vi "LU20_krio_main__.vi"() -> ()   [LabVIEW 2015]
doc: "Программа мониторинга температуры ОГ-1000"
uses:
  <vilib>/NI/Modbus Library/API/Master/Modbus Master.lvclass
  <vilib>/Utility/error.llb/DialogType.ctl
panel:
  out "Связь с блоком":bool
  in  "Tab Control":enum32{"ИЗМЕРЕНИЯ [ K ]", "НАСТРОЙКИ"}(tab)
  out "R2":dbl format="%.2f"
  out "R1":dbl format="%.2f"
  in  "2_ch_visible":bool=TRUE
  in  "1_ch_visible":bool=TRUE
  out "T2":dbl format="%.2f"
  out "T1":dbl format="%.2f"
  out "Путь к файлу с коэф.":path
  in  "Пароль":string
  in  "настр. коэфф.":bool caption="Disconn"
  in  "Coeff_cl_ch2":T1={"k1"=31.9101907935109921, "k2"=-399.867376562207937, "k3"=2119.32627579197288, "k4"=-5531.15447566658258, "k5"=7772.21873644739389, "k6"=-5292.23886113613844, "k7"=1613.2211984321475, "R0"=1613.2211984321475} caption="T2" {"R0" format="%#_16g"; "k7" format="%#_16g"; "k6" format="%#_16g"; "k5" format="%#_16g"; "k4" format="%#_16g"; "k3" format="%#_16g"; "k2" format="%#_16g"; "k1" format="%#_16g"}
  in  "load_coeff.":bool caption="Disconn"
  in  "save_coeff.":bool caption="Disconn"
  in  "xScale -":bool
  in  "xScale +":bool
  out "мин.":string="1"
  in  "Добавить время":dbl(ring)=300.0 items=["10 сек."=10.0, "1 мин."=60.0, "5 мин."=300.0, "20 мин."=1200.0]
  out "часы":string="0"
  out "сек.":string="0"
  in  "stop":bool
  in  "Coeff_cl_ch1":T1 caption="T1" {"R0" format="%#_16g"; "k7" format="%#_16g"; "k6" format="%#_16g"; "k5" format="%#_16g"; "k4" format="%#_16g"; "k3" format="%#_16g"; "k2" format="%#_16g"; "k1" format="%#_16g"}
  in  "GraphLookB":bool
  in  "Т min":dbl=4.0 min=-10.0 max=350.0 step=0.1
  in  "Т max":dbl=350.0 min=2.0 max=500.0 step=0.1
  in  "Autoscale":bool=TRUE
  in  "IP":string
  in  "Порт":u16
  out "Сутки":string
  in  "Запись в файл":bool
  out "Path":string
  out "File header exist?":bool caption="Disconn"
  in  "ADC_dyn_range":T2(ring)=enum."± 0.625 В"
  out "refnum out":refnum<file>
  out "Graphs T":dynamicdata(graph) caption="ИЗМЕРЕНИЯ ТЕМПЕРАТУРЫ, К"
  out "Связь":refnum<class "Modbus Master.lvclass">
  in  "Buf_size":u8=1 min=1 max=128
  in  "SPS":T3(ring)
  out "Расположение файла":path
  # "Соед."
  # "K"
  # "K"
  # "Ом"
  # "Ом"
  # ":"
  # ":"
  # "id 102"
  # "Шкала Т"
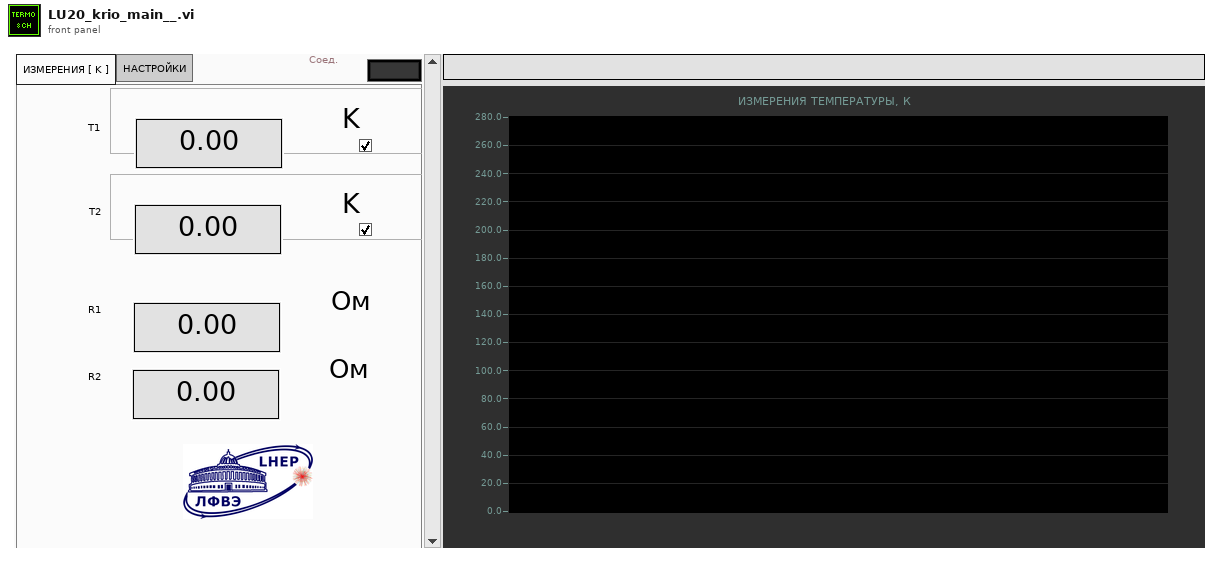
[diagram p1: front panel]
types:
  T1 = cluster{"k1":ext, "k2":ext, "k3":ext, "k4":ext, "k5":ext, "k6":ext, "k7":ext, "R0":ext}
  T2 = enum16{"± 5 В", "± 2.5 В", "± 1.25 В", "± 0.625 В", "± 312.5 мВ", "± 156.25 мВ", "± 78.125 мВ"}
  T3 = enum16{"2,5 SPS", "5 SPS", "10 SPS", "25 SPS", "50 SPS", "100 SPS", "500 SPS", "1 kSPS"}
  T4 = typedef "DialogType.ctl" = u16
  T5 = enum8{"Enabled", "Disabled", "Disabled and Grayed Out"}
  T6 = typedef "LVDateTimeRec.ctl" = cluster{"fractional second":dbl, "second":i32, "minute":i32, "hour":i32, "day of month":i32, "month":i32, "year":i32, "day of week":i32, "day of year":i32, "DST":i32}
  T7 = enum16{"open", "replace", "create", "open or create", "replace or create", "replace or create with confirmation"}
  T8 = cluster{"k1":ext, "k2":ext, "k3":ext, "k4":ext, "k5":ext, "k6":ext, "k7":ext, "R":ext}
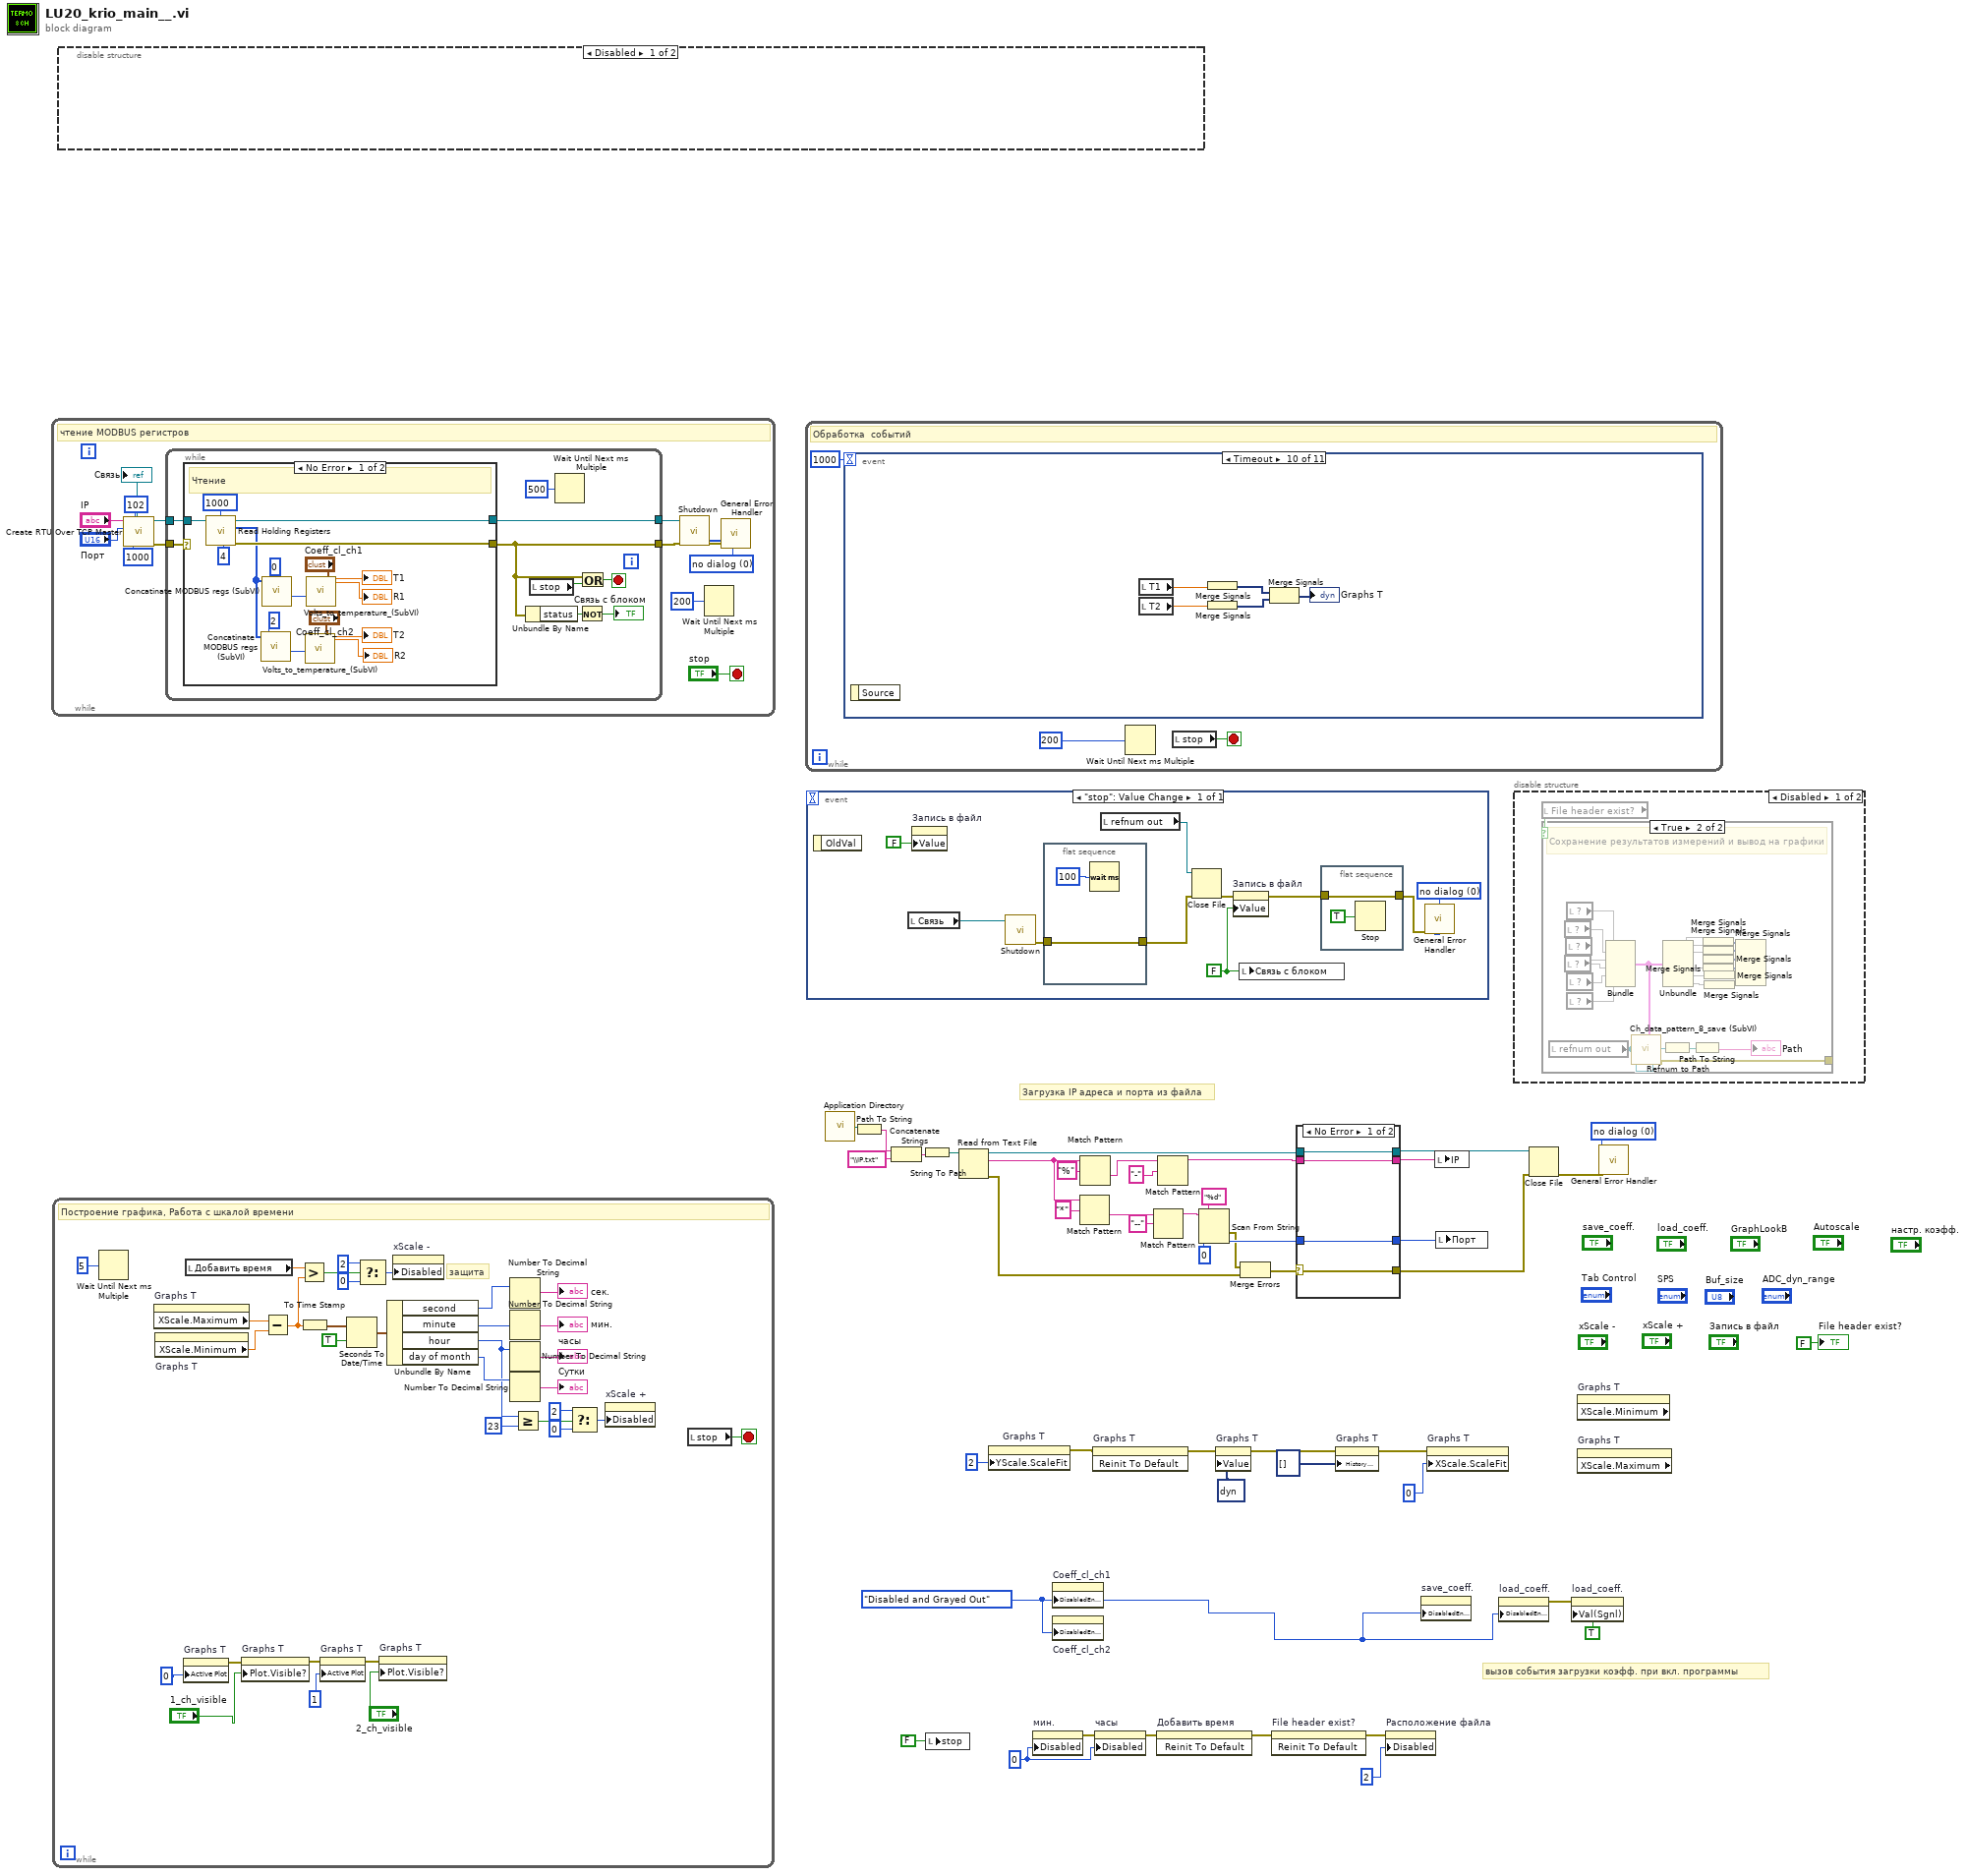
[diagram p0: block diagram]
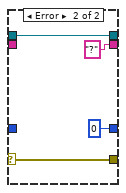
[diagram p2: hidden frame]
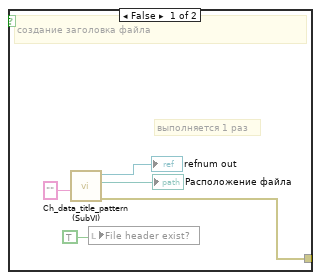
[diagram p4: hidden frame]
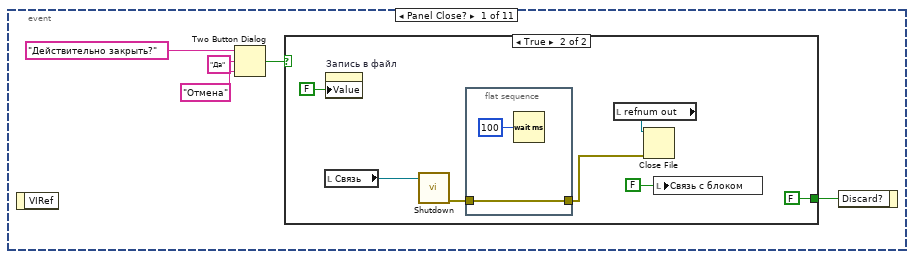
[diagram p6: hidden frame]
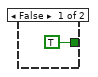
[diagram p7: hidden frame]
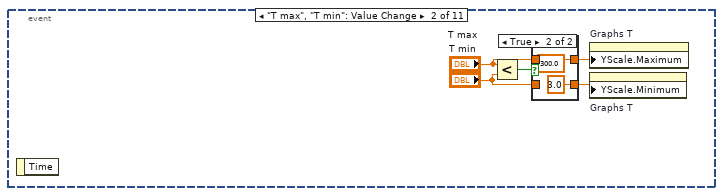
[diagram p8: hidden frame]
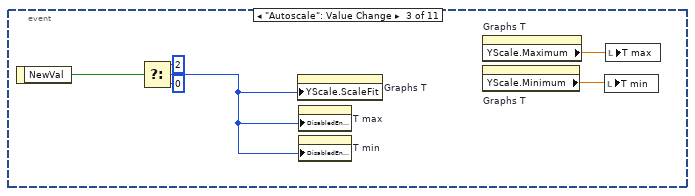
[diagram p10: hidden frame]
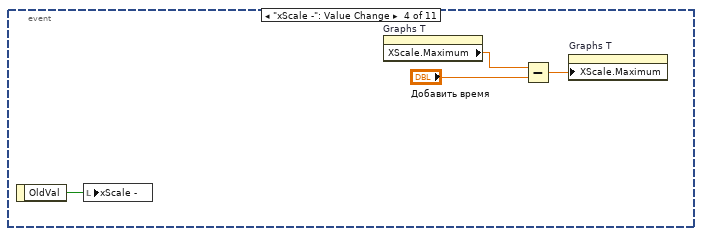
[diagram p11: hidden frame]
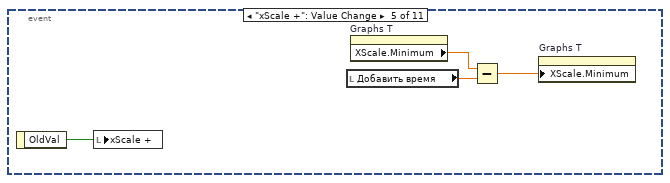
[diagram p12: hidden frame]
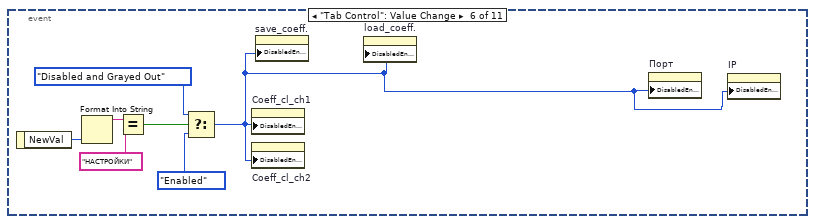
[diagram p13: hidden frame]
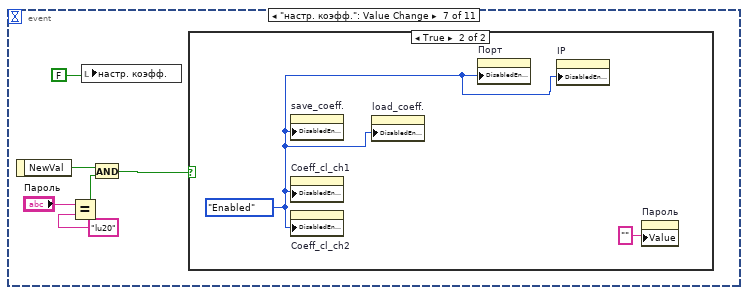
[diagram p14: hidden frame]
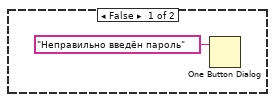
[diagram p15: hidden frame]
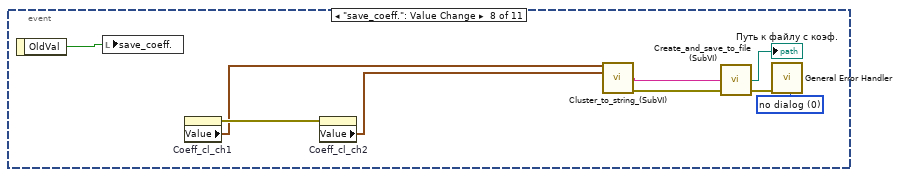
[diagram p16: hidden frame]
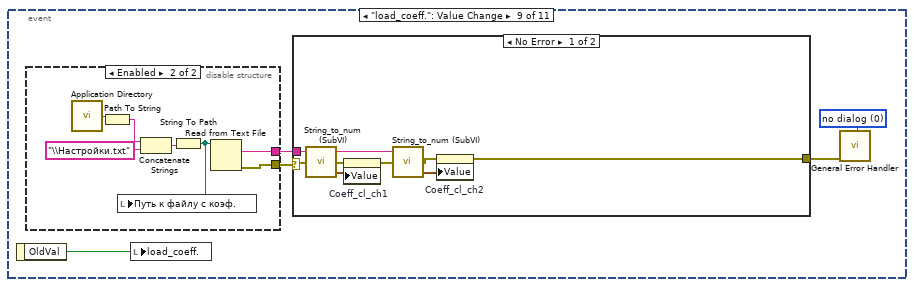
[diagram p17: hidden frame]
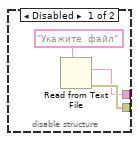
[diagram p18: hidden frame]
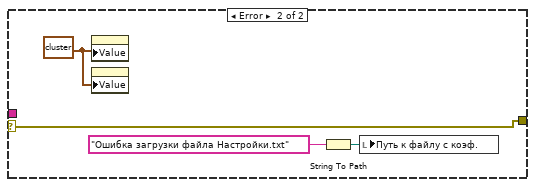
[diagram p19: hidden frame]
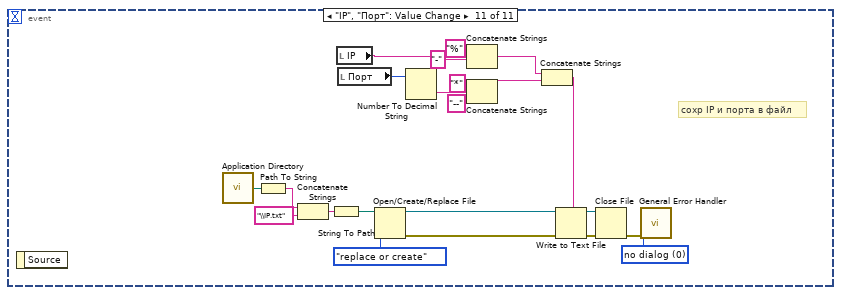
[diagram p20: hidden frame]
diagram:
  w10 = T4 0 items=["no dialog", "OK message", "continue or stop message", "OK message + warnings", "continue/stop + warnings"] ("type of dialog (OK msg:1)")
  w38 = T5."Disabled and Grayed Out" ("Disabled")
  w45 = u8 0 ("Disabled")
  # "Загрузка IP адреса и порта из файла"
  # "вызов события загрузки коэфф. при вкл. программы"
  n1 = while {
    stop <- "stop" stop-if-true
    w47 = T4 0 items=["no dialog", "OK message", "continue or stop message", "OK message + warnings", "continue/stop + warnings"] ("type of dialog (OK msg:1)")
    # "чтение MODBUS регистров"
    n2 = call "Create RTU Over TCP Master.vi"("unit ID"=u8 102 ("ID"), "connect timeout ms"=1000, "port (502)"="Порт", "address"="IP") -> ("error out"=w51:errorcluster, "TCP master instance"=w52:refnum<class "Modbus Master.lvclass">)  [unwired: 6 in]
    "Связь" <- w52
    n3 = while {
      tunnel: w52 -> [w67]
      tunnel: w51 -> [w66]
      tunnel: [w60] -> w50
      tunnel: [w65] -> w49
      stop <- w63 stop-if-true
      n4 = case shown="No Error" w66 {
        selector: w66 -> [_ w84]
        tunnel: w67 -> [w81 w85]
        tunnel: [w78 w84] -> w60
        tunnel: [w80 w85] -> w65
        frame No Error {
          # "Чтение"
          n5 = call-dynamic "Read Holding Registers.vi"("number of inputs"=u16 4, "starting address"=u16 1000, "Modbus master in"=w81) -> ("error out"=w78:errorcluster, "register values"=w72:u16[], "Modbus master out"=w80:refnum<class "Modbus Master.lvclass">)  [unwired: 6 in]
          n6 = call "Concatinate MODBUS regs (SubVI).vi"("LSB reg num"=u16 2, "registers array in"=w72) -> ("register data"=w74:i32)  [unwired: 8 in, 1 out]
          n7 = call "Concatinate MODBUS regs (SubVI).vi"("LSB reg num"=u16 0, "registers array in"=w72) -> ("register data"=w76:i32)  [unwired: 8 in, 1 out]
          n8 = call "Volts_to_temperature_(SubVI).vi"("Resistance"=w74, "koeff. cluster"="Coeff_cl_ch2") -> ("T solvation"=→"T2":dbl, "meas_voltage"=→"R2":dbl)  [unwired: 21 in, 3 out]
          n9 = call "Volts_to_temperature_(SubVI).vi"("Resistance"=w76, "koeff. cluster"="Coeff_cl_ch1") -> ("T solvation"=→"T1":dbl, "meas_voltage"=→"R1":dbl)  [unwired: 21 in, 3 out]
        }
        frame Error {
        }
      }
      n10 = Unbundle By Name(w60) -> ("status"=w62:bool)
      n11 = local read "stop"() -> (w64:bool)
      n12 = Wait Until Next ms Multiple(millisecond multiple=u32 500) -> ()  [unwired: 1 out]
      n13 = Not(x=w62) -> (.not. x?=→"Связь с блоком":bool)
      n14 = Or(x=w60, y=w64) -> (x .or. y?=w63:bool)
    }
    n15 = call-dynamic "Shutdown.vi"("error in"=w50, "Modbus master in"=w49) -> ("error out"=w48:errorcluster)  [unwired: 9 in]
    n16 = Wait Until Next ms Multiple(millisecond multiple=u32 200) -> ()  [unwired: 1 out]
    n17 = call <vilib>:"General Error Handler.vi"("type of dialog (OK msg:1)"=w47, "error in (no error)"=w48) -> ()  [unwired: 1 in, 13 out]
  }
  n18 = while {
    stop <- w118 stop-if-true
    # "защита"
    # "Построение графика, Работа с шкалой времени"
    n19 = Wait Until Next ms Multiple(millisecond multiple=u32 5) -> ()  [unwired: 1 out]
    n20 = property on="Graphs T" class="WFChart (strict)"() -> ("XScale.Maximum"=w94:dbl)  [unwired: 2 in, 2 out]
    n21 = property on="Graphs T" class="WFChart (strict)"() -> ("XScale.Minimum"=w93:dbl)  [unwired: 2 in, 2 out]
    n22 = property on="Graphs T" class="WFChart (strict)"("Active Plot"=u32 0) -> (error out=w86:errorcluster)  [unwired: 2 in, 1 out]
    n23 = local read "Добавить время"() -> (w117:dbl)
    n24 = property on="Graphs T" class="WFChart (strict)"(error in=w86, "Plot.Visible?"="1_ch_visible") -> (error out=w91:errorcluster)  [unwired: 1 in, 1 out]
    n25 = Subtract(x=w94, y=w93) -> (x-y=w107:dbl)
    n26 = Greater?(x=w117, y=w107) -> (0:w100:bool)
    n27 = To Time Stamp(1:w107) -> (0:w115:timestamp)
    n28 = property on="Graphs T" class="WFChart (strict)"(error in=w91, "Active Plot"=u32 1) -> (error out=w89:errorcluster)  [unwired: 1 in, 1 out]
    n29 = Seconds To Date/Time(time stamp (now)=w115, to UTC (F)=TRUE) -> (date time rec=w114:T6)
    n30 = Select(t=u8 2 ("Disabled"), s=w100, f=u8 0 ("Disabled")) -> (s? t:f=w103:u8)
    n31 = property on="Graphs T" class="WFChart (strict)"(error in=w89, "Plot.Visible?"="2_ch_visible") -> ()  [unwired: 1 in, 2 out]
    n32 = Unbundle By Name(w114) -> ("second"=w113:i32, "minute"=w112:i32, "hour"=w105:i32, "day of month"=w111:i32)
    n33 = property on="xScale -" class="Bool (strict)"("Disabled"=w103) -> ()  [unwired: 2 in, 2 out]
    n34 = Number To Decimal String(number=w113) -> (decimal integer string=→"сек.":string)  [unwired: 1 out]
    n35 = Number To Decimal String(number=w112) -> (decimal integer string=→"мин.":string)  [unwired: 1 out]
    n36 = Number To Decimal String(number=w105) -> (decimal integer string=→"часы":string)  [unwired: 1 out]
    n37 = Number To Decimal String(number=w111) -> (decimal integer string=→"Сутки":string)  [unwired: 1 out]
    n38 = Greater Or Equal?(x=w105, y=23) -> (x >= y?=w96:bool)
    n39 = Select(t=u8 2 ("Disabled"), s=w96, f=u8 0 ("Disabled")) -> (s? t:f=w99:u8)
    n40 = property on="xScale +" class="Bool (strict)"("Disabled"=w99) -> ()  [unwired: 2 in, 2 out]
    n41 = local read "stop"() -> (w118:bool)
  }
  n42 = disable-structure shown="Disabled" {
    frame Disabled {
    }
    frame Enabled {
    }
  }
  n43 = while {
    stop <- w120 stop-if-true
    # "Обработка  событий"
    n44 = event shown="[9] Timeout" {
      selector: _ -> [_ _ _ _ _ _ _ _ _ _ _]
      dyn-events: _ -> [_ _ _ _ _ _ _ _ _ _ _]
      timeout: 1000 -> [_ _ _ _ _ _ _ _ _ _ _]
      event Panel Close? {
        n45 = event-data() -> ()  [unwired: 2 out]
        n46 = Two Button Dialog(message="Действительно закрыть?", 1:"Отмена" ("T button name (\"OK\")"), 2:"Да" ("T button name (\"OK\")")) -> (T button?=w126:bool)
        n47 = case shown="True" w126 {
          tunnel: [TRUE ("Discard?") FALSE ("Discard?")] -> w122
          frame False {
          }
          frame True {
            n48 = local read "Связь"() -> (w131:refnum<class "Modbus Master.lvclass">)
            n49 = property on="Запись в файл" class="Bool (strict)"("Value"=FALSE ("Запись в файл")) -> ()  [unwired: 2 in, 2 out]
            n50 = call-dynamic "Shutdown.vi"("Modbus master in"=w131) -> ("error out"=w130:errorcluster)  [unwired: 10 in]
            n51 = flat-sequence {
              tunnel: w130 -> [w135]
              tunnel: [w135] -> w129
              frame #0 {
                n52 = Wait (ms)(milliseconds to wait=u32 100) -> ()  [unwired: 1 out]
              }
            }
            n53 = local read "refnum out"() -> (w133:refnum<file>)
            n54 = Close File(refnum=w133, error in=w129) -> ()  [unwired: 2 out]
            n55 = local write "Связь с блоком"(FALSE ("Связь с блоком 4")) -> ()
          }
        }
        n56 = event-data("Discard?"=w122) -> ()  [unwired: 1 in, 1 out]
      }
      event "Т max", "Т min": Value Change {
        n57 = event-data() -> ()  [unwired: 2 out]
        n58 = Less?(x="Т max", y="Т min") -> (x < y?=w141:bool)
        n59 = case shown="True" w141 {
          tunnel: [w142 300.0 ("x+1")] -> w139
          tunnel: [w143 3.0 ("x+1")] -> w140
          tunnel: "Т max" -> [w142 _]
          tunnel: "Т min" -> [w143 _]
          frame False {
          }
          frame True {
          }
        }
        n60 = property on="Graphs T" class="WFChart (strict)"("YScale.Maximum"=w139) -> ()  [unwired: 2 in, 2 out]
        n61 = property on="Graphs T" class="WFChart (strict)"("YScale.Minimum"=w140) -> ()  [unwired: 2 in, 2 out]
      }
      event "Autoscale": Value Change {
        n62 = event-data() -> ("NewVal"=w146:bool)  [unwired: 1 out]
        n63 = Select(t=u8 2 ("Y Scale.Scale Fit"), s=w146, f=u8 0 ("Y Scale.Scale Fit")) -> (s? t:f=w149:u8)
        n64 = property on="Graphs T" class="WFChart (strict)"("YScale.ScaleFit"=w149) -> ()  [unwired: 2 in, 2 out]
        n65 = property on="Т max" class="DigNum (strict)"("DisabledEnum"=w149) -> ()  [unwired: 2 in, 2 out]
        n66 = property on="Т min" class="DigNum (strict)"("DisabledEnum"=w149) -> ()  [unwired: 2 in, 2 out]
        n67 = property on="Graphs T" class="WFChart (strict)"() -> ("YScale.Maximum"=w151:dbl)  [unwired: 2 in, 2 out]
        n68 = property on="Graphs T" class="WFChart (strict)"() -> ("YScale.Minimum"=w150:dbl)  [unwired: 2 in, 2 out]
        n69 = local write "Т min"(w150) -> ()
        n70 = local write "Т max"(w151) -> ()
      }
      event "xScale -": Value Change {
        n71 = event-data() -> ("OldVal"=w155:bool)  [unwired: 1 out]
        n72 = local write "xScale -"(w155) -> ()
        n73 = property on="Graphs T" class="WFChart (strict)"() -> ("XScale.Maximum"=w153:dbl)  [unwired: 2 in, 2 out]
        n74 = Subtract(x=w153, y="Добавить время") -> (x-y=w152:dbl)
        n75 = property on="Graphs T" class="WFChart (strict)"("XScale.Maximum"=w152) -> ()  [unwired: 2 in, 2 out]
      }
      event "xScale +": Value Change {
        n76 = event-data() -> ("OldVal"=w159:bool)  [unwired: 1 out]
        n77 = local write "xScale +"(w159) -> ()
        n78 = local read "Добавить время"() -> (w158:dbl)
        n79 = property on="Graphs T" class="WFChart (strict)"() -> ("XScale.Minimum"=w157:dbl)  [unwired: 2 in, 2 out]
        n80 = Subtract(x=w157, y=w158) -> (x-y=w156:dbl)
        n81 = property on="Graphs T" class="WFChart (strict)"("XScale.Minimum"=w156) -> ()  [unwired: 2 in, 2 out]
      }
      event "Tab Control": Value Change {
        n82 = event-data() -> ("NewVal"=w166:enum32{"ИЗМЕРЕНИЯ [ K ]", "НАСТРОЙКИ"})  [unwired: 1 out]
        n83 = Format Into String(w166) -> (resulting string=w165:string)  [unwired: 3 in, 1 out]
        n84 = Equal?(x=w165, y="НАСТРОЙКИ") -> (x = y?=w163:bool)
        n85 = Select(t=T5."Disabled and Grayed Out" ("Disabled"), s=w163, f=T5."Enabled" ("Disabled")) -> (s? t:f=w160:T5)
        n86 = property on="Coeff_cl_ch1" class="Clust (strict)"("DisabledEnum"=w160) -> ()  [unwired: 2 in, 2 out]
        n87 = property on="Coeff_cl_ch2" class="Clust (strict)"("DisabledEnum"=w160) -> ()  [unwired: 2 in, 2 out]
        n88 = property on="save_coeff." class="Bool (strict)"("DisabledEnum"=w160) -> ()  [unwired: 2 in, 2 out]
        n89 = property on="load_coeff." class="Bool (strict)"("DisabledEnum"=w160) -> ()  [unwired: 2 in, 2 out]
        n90 = property on="Порт" class="DigNum (strict)"("DisabledEnum"=w160) -> ()  [unwired: 2 in, 2 out]
        n91 = property on="IP" class="Str"("DisabledEnum"=w160) -> ()  [unwired: 2 in, 2 out]
      }
      event "настр. коэфф.": Value Change {
        n92 = event-data() -> ("NewVal"=w172:bool)  [unwired: 1 out]
        n93 = Equal?(x="Пароль", y="lu20") -> (x = y?=w169:bool)
        n94 = local write "настр. коэфф."(FALSE ("насстр. коэфф.")) -> ()
        n95 = And(x=w172, y=w169) -> (x .and. y?=w168:bool)
        n96 = case shown="True" w168 {
          frame False {
            n97 = One Button Dialog(message="Неправильно введён пароль") -> ()  [unwired: 1 in, 1 out]
          }
          frame True {
            w174 = T5."Enabled" ("Disabled")
            n98 = property on="save_coeff." class="Bool (strict)"("DisabledEnum"=w174) -> ()  [unwired: 2 in, 2 out]
            n99 = property on="Coeff_cl_ch1" class="Clust (strict)"("DisabledEnum"=w174) -> ()  [unwired: 2 in, 2 out]
            n100 = property on="Coeff_cl_ch2" class="Clust (strict)"("DisabledEnum"=w174) -> ()  [unwired: 2 in, 2 out]
            n101 = property on="load_coeff." class="Bool (strict)"("DisabledEnum"=w174) -> ()  [unwired: 2 in, 2 out]
            n102 = property on="Порт" class="DigNum (strict)"("DisabledEnum"=w174) -> ()  [unwired: 2 in, 2 out]
            n103 = property on="IP" class="Str"("DisabledEnum"=w174) -> ()  [unwired: 2 in, 2 out]
            n104 = property on="Пароль" class="Str"("Value"="" ("Пароль")) -> ()  [unwired: 2 in, 2 out]
          }
        }
      }
      event "save_coeff.": Value Change {
        w178 = T4 0 items=["no dialog", "OK message", "continue or stop message", "OK message + warnings", "continue/stop + warnings"] ("type of dialog (OK msg:1)")
        n105 = event-data() -> ("OldVal"=w184:bool)  [unwired: 1 out]
        n106 = local write "save_coeff."(w184) -> ()
        n107 = property on="Coeff_cl_ch1" class="Clust (strict)"() -> (error out=w183:errorcluster, "Value"=w182:T1)  [unwired: 2 in, 1 out]
        n108 = property on="Coeff_cl_ch2" class="Clust (strict)"(error in=w183) -> ("Value"=w181:T1)  [unwired: 1 in, 2 out]
        n109 = call "Cluster_to_string_(SubVI).vi"("input cluster 1"=w182, "input cluster 2"=w181) -> ("string of coefficients"=w176:string, "error out"=w180:errorcluster)  [unwired: 12 in]
        n110 = call "Create_and_save_to_file (SubVI).vi"("input string"=w176, "error in"=w180) -> ("Текущее расположение файла"=→"Путь к файлу с коэф.":path, "error out"=w179:errorcluster)  [unwired: 4 in]
        n111 = call <vilib>:"General Error Handler.vi"("type of dialog (OK msg:1)"=w178, "error in (no error)"=w179) -> ()  [unwired: 9 in, 5 out]
      }
      event "load_coeff.": Value Change {
        w187 = T4 0 items=["no dialog", "OK message", "continue or stop message", "OK message + warnings", "continue/stop + warnings"] ("type of dialog (OK msg:1)")
        n112 = event-data() -> ("OldVal"=w189:bool)  [unwired: 1 out]
        n113 = disable-structure shown="Enabled" {
          disable-tunnel: [w192 w195] -> w186
          disable-tunnel: [w191 w196] -> w188
          frame Disabled {
            n114 = Read from Text File(prompt (Open existing file)="Укажите  файл") -> (text=w191:string, cancelled=w193:bool, error out=w192:errorcluster)  [unwired: 3 in, 1 out]
          }
          frame Enabled {
            n115 = call <vilib>:"Application Directory.vi"() -> ("Application Directory"=w200:path)
            n116 = Path To String(path=w200) -> (string=w199:string)
            n117 = Concatenate Strings(w199, "\\Настройки.txt" ("prompt (Open existing file)")) -> (w198:string)
            n118 = String To Path(string=w198) -> (path=w194:path)
            n119 = local write "Путь к файлу с коэф."(w194) -> ()
            n120 = Read from Text File(file (use dialog)=w194) -> (text=w196:string, error out=w195:errorcluster)  [unwired: 3 in, 2 out]
          }
        }
        n121 = local write "load_coeff."(w189) -> ()
        n122 = case shown="No Error" w186 {
          selector: w186 -> [w202 w210]
          tunnel: w188 -> [w209 _]
          tunnel: [w201 w210] -> w185
          frame No Error {
            n123 = call "String_to_num (SubVI).vi"("String in"=w209, "error in"=w202) -> ("Rest of string OUT"=w206:string, "error out"=w207:errorcluster, "output cluster \nof coefficients"=w208:T8)  [unwired: 5 in]
            n124 = property on="Coeff_cl_ch1" class="Clust (strict)"(error in=w207, "Value"=w208) -> (error out=w205:errorcluster)  [unwired: 1 in, 1 out]
            n125 = call "String_to_num (SubVI).vi"("String in"=w206, "error in"=w205) -> ("error out"=w204:errorcluster, "output cluster \nof coefficients"=w203:T8)  [unwired: 5 in, 1 out]
            n126 = property on="Coeff_cl_ch2" class="Clust (strict)"(error in=w204, "Value"=w203) -> (error out=w201:errorcluster)  [unwired: 1 in, 1 out]
          }
          frame Error {
            w211 = T1 {"k1"=0.0, "k2"=0.0, "k3"=0.0, "k4"=0.0, "k5"=0.0, "k6"=0.0, "k7"=0.0, "R0"=0.0} ("Coeff_cl_ch1")
            n127 = property on="Coeff_cl_ch1" class="Clust (strict)"("Value"=w211) -> ()  [unwired: 2 in, 2 out]
            n128 = property on="Coeff_cl_ch2" class="Clust (strict)"("Value"=w211) -> ()  [unwired: 2 in, 2 out]
            n129 = String To Path(string="Ошибка загрузки файла Настройки.txt") -> (path=w213:path)
            n130 = local write "Путь к файлу с коэф."(w213) -> ()
          }
        }
        n131 = call <vilib>:"General Error Handler.vi"("type of dialog (OK msg:1)"=w187, "error in (no error)"=w185) -> ()  [unwired: 9 in, 5 out]
      }
      event Timeout {
        n132 = event-data() -> ()  [unwired: 2 out]
        n133 = local read "T1"() -> (w215:dbl)
        n134 = local read "T2"() -> (w214:dbl)
        n135 = Merge Signals(w215) -> (w218:dynamicdata)
        n136 = Merge Signals(w214) -> (w217:dynamicdata)
        n137 = Merge Signals(w218, w217) -> (→"Graphs T":dynamicdata)
      }
      event "IP", "Порт": Value Change {
        w222 = T4 0 items=["no dialog", "OK message", "continue or stop message", "OK message + warnings", "continue/stop + warnings"] ("type of dialog (OK msg:1)")
        # "сохр IP и порта в файл"
        n138 = event-data() -> ()  [unwired: 2 out]
        n139 = call <vilib>:"Application Directory.vi"() -> ("Application Directory"=w240:path)
        n140 = Path To String(path=w240) -> (string=w239:string)
        n141 = Concatenate Strings(w239, "\\IP.txt" ("prompt (Open existing file)")) -> (w238:string)
        n142 = String To Path(string=w238) -> (path=w223:path)
        n143 = local read "IP"() -> (w236:string)
        n144 = local read "Порт"() -> (w235:u16)
        n145 = Open/Create/Replace File(file path (use dialog)=w223, operation (0:open)=T7."replace or create") -> (refnum out=w226:refnum<file>, error out=w225:errorcluster)  [unwired: 1 in, 4 out]
        n146 = Number To Decimal String(number=w235) -> (decimal integer string=w231:string)  [unwired: 1 in]
        n147 = Concatenate Strings("%" ("string"), w236, "-" ("string")) -> (w232:string)
        n148 = Concatenate Strings("*" ("string"), w231, "--" ("string")) -> (w233:string)
        n149 = Concatenate Strings(w232, w233) -> (w234:string)
        n150 = Write to Text File(file (use dialog)=w226, text=w234, error in=w225) -> (refnum out=w228:refnum<file>, error out=w227:errorcluster)  [unwired: 2 out]
        n151 = Close File(refnum=w228, error in=w227) -> (error out=w221:errorcluster)  [unwired: 1 out]
        n152 = call <vilib>:"General Error Handler.vi"("type of dialog (OK msg:1)"=w222, "error in (no error)"=w221) -> ()  [unwired: 1 in, 13 out]
      }
    }
    n153 = Wait Until Next ms Multiple(millisecond multiple=u32 200) -> ()  [unwired: 1 out]
    n154 = local read "stop"() -> (w120:bool)
  }
  n155 = event shown="[0] \"stop\": Value Change" {
    selector: _ -> [_]
    dyn-events: _ -> [_]
    timeout: _ -> [_]
    event "stop": Value Change {
      w244 = T4 0 items=["no dialog", "OK message", "continue or stop message", "OK message + warnings", "continue/stop + warnings"] ("type of dialog (OK msg:1)")
      w241 = FALSE ("Запись в файл")
      n156 = event-data() -> ()  [unwired: 1 in, 1 out]
      n157 = local read "Связь"() -> (w246:refnum<class "Modbus Master.lvclass">)
      n158 = property on="Запись в файл" class="Bool (strict)"("Value"=FALSE ("Запись в файл")) -> ()  [unwired: 2 in, 2 out]
      n159 = call-dynamic "Shutdown.vi"("Modbus master in"=w246) -> ("error out"=w245:errorcluster)  [unwired: 10 in]
      n160 = flat-sequence {
        tunnel: w245 -> [w253]
        tunnel: [w253] -> w242
        frame #0 {
          n161 = Wait (ms)(milliseconds to wait=u32 100) -> ()  [unwired: 1 out]
        }
      }
      n162 = local read "refnum out"() -> (w249:refnum<file>)
      n163 = Close File(refnum=w249, error in=w242) -> (error out=w248:errorcluster)  [unwired: 1 out]
      n164 = property on="Запись в файл" class="Bool (strict)"(error in=w248, "Value"=w241) -> (error out=w247:errorcluster)  [unwired: 1 in, 1 out]
      n165 = local write "Связь с блоком"(w241) -> ()
      n166 = flat-sequence {
        tunnel: w247 -> [w252]
        tunnel: [w252] -> w243
        frame #0 {
          n167 = Stop(stop? (T)=TRUE) -> ()
        }
      }
      n168 = call <vilib>:"General Error Handler.vi"("error in (no error)"=w243, "[exception action] (none:0)"=w244) -> ()  [unwired: 2 in, 12 out]
    }
  }
  n169 = call <vilib>:"Application Directory.vi"() -> ("Application Directory"=w29:path)
  n170 = Path To String(path=w29) -> (string=w30:string)
  n171 = Concatenate Strings(w30, "\\IP.txt" ("prompt (Open existing file)")) -> (w31:string)
  n172 = String To Path(string=w31) -> (path=w33:path)
  n173 = local write "stop"(FALSE ("Boolean")) -> ()
  n174 = Read from Text File(file (use dialog)=w33) -> (refnum out=w22:refnum<file>, text=w35:string, error out=w1:errorcluster)  [unwired: 3 in, 1 out]
  n175 = property on="Graphs T" class="WFChart (strict)"("YScale.ScaleFit"=u8 2 ("Y Scale.Scale Fit")) -> (error out=w9:errorcluster)  [unwired: 2 in, 1 out]
  n176 = property on="мин." class="Str"("Disabled"=w45) -> (error out=w44:errorcluster)  [unwired: 2 in, 1 out]
  n177 = property on="Coeff_cl_ch1" class="Clust (strict)"("DisabledEnum"=w38) -> ()  [unwired: 2 in, 2 out]
  n178 = property on="Coeff_cl_ch2" class="Clust (strict)"("DisabledEnum"=w38) -> ()  [unwired: 2 in, 2 out]
  n179 = Match Pattern(string=w35, regular expression="*") -> (after substring=w14:string)  [unwired: 1 in, 3 out]
  n180 = Match Pattern(string=w35, regular expression="%") -> (after substring=w28:string)  [unwired: 1 in, 3 out]
  n181 = invoke on="Graphs T" class="WFChart (strict)" method="Reinit To Default"(error in=w9) -> (error out=w5:errorcluster)  [unwired: 2 in, 2 out]
  n182 = property on="часы" class="Str"(error in=w44, "Disabled"=w45) -> (error out=w43:errorcluster)  [unwired: 1 in, 1 out]
  n183 = Match Pattern(string=w14, regular expression="--" ("string")) -> (before substring=w13:string)  [unwired: 1 in, 3 out]
  n184 = invoke on="Добавить время" class="Ring (strict)" method="Reinit To Default"(error in=w43) -> (error out=w41:errorcluster)  [unwired: 2 in, 2 out]
  n185 = Match Pattern(string=w28, regular expression="-" ("string")) -> (before substring=w27:string)  [unwired: 1 in, 3 out]
  n186 = Scan From String(format string="%d", input string=w13, default 1=u16 0 ("default value 1")) -> (error out=w12:errorcluster, output 1=w26:u16)  [unwired: 2 in, 2 out]
  n187 = property on="Graphs T" class="WFChart (strict)"(error in=w5, "Value"=dynamicdata [{"t0"=timestamp(3465273261.7246556 s since 1904-01-01), "dt"=1.0, "Y"=[0.1931097262457384]}, {"t0"=timestamp(3465273261.7246556 s since 1904-01-01), "dt"=1.0, "Y"=[0.3594116459482981]}, {"t0"=timestamp(3465273261.7246556 s since 1904-01-01), "dt"=1.0, "Y"=[0.8898205452798131]}, {"t0"=timestamp(3465273261.7246556 s since 1904-01-01), "dt"=1.0, "Y"=[0.747699236883661]}] ("Graphs")) -> (error out=w6:errorcluster)  [unwired: 1 in, 1 out]
  n188 = Merge Errors(w12, w1) -> (w25:errorcluster)
  n189 = invoke on="File header exist?" class="Bool (strict)" method="Reinit To Default"(error in=w41) -> (error out=w42:errorcluster)  [unwired: 2 in, 2 out]
  n190 = case shown="No Error" w25 {
    selector: w25 -> [w256 w259]
    tunnel: w27 -> [w258 _]
    tunnel: w26 -> [w257 _]
    tunnel: [w258 "?"] -> w24
    tunnel: [w257 u16 0 ("default value 1")] -> w23
    tunnel: w22 -> [w255 w260]
    tunnel: [w255 w260] -> w21
    tunnel: [w256 w259] -> w20
    frame No Error {
    }
    frame Error {
    }
  }
  n191 = property on="Graphs T" class="WFChart (strict)"(error in=w6, "History Data"=dynamicdata[] []) -> (error out=w3:errorcluster)  [unwired: 1 in, 1 out]
  n192 = property on="Расположение файла" class="Path"(error in=w42, "Disabled"=u8 2) -> ()  [unwired: 1 in, 2 out]
  n193 = property on="save_coeff." class="Bool (strict)"("DisabledEnum"=w38) -> ()  [unwired: 2 in, 2 out]
  n194 = property on="Graphs T" class="WFChart (strict)"(error in=w3, "XScale.ScaleFit"=u8 0 ("Y Scale.Scale Fit")) -> ()  [unwired: 1 in, 2 out]
  n195 = local write "IP"(w24) -> ()
  n196 = local write "Порт"(w23) -> ()
  n197 = property on="load_coeff." class="Bool (strict)"("DisabledEnum"=w38) -> (error out=w36:errorcluster)  [unwired: 2 in, 1 out]
  n198 = disable-structure shown="Disabled" {
    frame Disabled {
      n199 = local read "File header exist?"() -> (w263:bool)
      n200 = case shown="True" w263 {
        tunnel: [w268 w291] -> _
        frame False {
          # "выполняется 1 раз"
          # "создание заголовка файла"
          n201 = call "Ch_data_title_pattern (SubVI).vi"("Единица измерений"="") -> ("error out"=w268:errorcluster, "Path"=→"Расположение файла":path, "Byte Stream File out"=→"refnum out":refnum<file>)  [unwired: 8 in]
          n202 = local write "File header exist?"(TRUE ("flag1")) -> ()
        }
        frame True {
          # "Сохранение результатов измерений и вывод на графики"
          n203 = local read "refnum out"() -> (w287:refnum<file>)
          n204 = local read item#-1() -> (w289)
          n205 = local read item#-1() -> (w275)
          n206 = local read item#-1() -> (w276)
          n207 = local read item#-1() -> (w290)
          n208 = local read item#-1() -> (w274)
          n209 = local read item#-1() -> (w271)
          n210 = Bundle(w290, w289, w276, w275, w274, w271) -> (w288:cluster{void, void, void, void, void, void})  [unwired: 1 in]
          n211 = call "Ch_data_pattern_8_save (SubVI).vi"("T Cluster"=w288, "file"=w287) -> ("error out"=w291:errorcluster)  [unwired: 25 in]
          n212 = Refnum to Path(1:w287) -> (0:w286:path)
          n213 = Unbundle(w288) -> (w280, w279, w278, w277, w272, w269)
          n214 = Path To String(path=w286) -> (string=→"Path":string)
          n215 = Merge Signals(w280) -> (w282:dynamicdata)
          n216 = Merge Signals(w279) -> (w283:dynamicdata)
          n217 = Merge Signals(w278) -> (w284:dynamicdata)
          n218 = Merge Signals(w277) -> (w281:dynamicdata)
          n219 = Merge Signals(w272) -> (w273:dynamicdata)
          n220 = Merge Signals(w269) -> (w270:dynamicdata)
          n221 = Merge Signals(w282, w283, w284, w281, w273, w270) -> ()  [unwired: 1 out]
        }
      }
    }
    frame Enabled {
    }
  }
  n222 = Close File(refnum=w21, error in=w20) -> (error out=w19:errorcluster)  [unwired: 1 out]
  n223 = property on="load_coeff." class="Bool (strict)"(error in=w36, "Val(Sgnl)"=TRUE ("Value (Signaling)")) -> ()  [unwired: 1 in, 2 out]
  n224 = property on="Graphs T" class="WFChart (strict)" props=["XScale", "Minimum"]() -> ()  [unwired: 2 in, 3 out]
  n225 = property on="Graphs T" class="WFChart (strict)" props=["XScale", "Maximum"]() -> ()  [unwired: 2 in, 3 out]
  n226 = call <vilib>:"General Error Handler.vi"("type of dialog (OK msg:1)"=w10, "error in (no error)"=w19) -> ()  [unwired: 1 in, 13 out]
  "File header exist?" <- FALSE ("flag1")
